vi "q4 character count.vi"() -> ()   [LabVIEW 2025]
panel:
  out "length without spaces":dbl
  out "text":string
  out "length":i32
  in  "Path":path
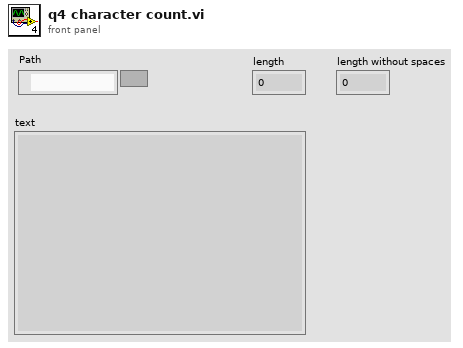
[diagram p1: front panel]
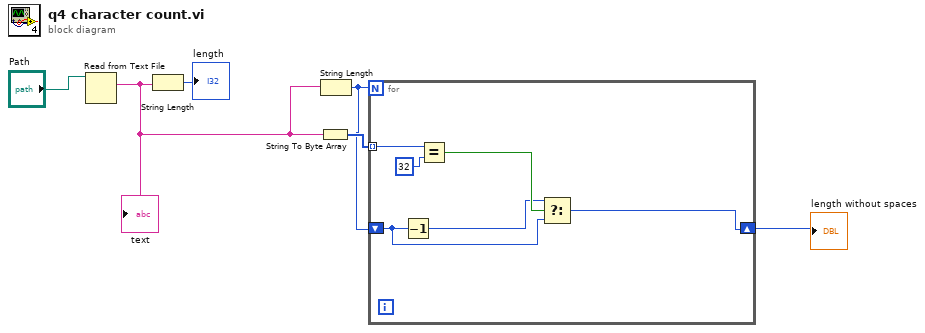
[diagram p0: block diagram]
diagram:
  n1 = Read from Text File(file (use dialog)="Path") -> (text=w2:string)  [unwired: 3 in, 3 out]
  "text" <- w2
  n2 = String Length(string=w2) -> (length=→"length":i32)
  n3 = String To Byte Array(string=w2) -> (unsigned byte array=w4:u8[])
  n4 = String Length(string=w2) -> (length=w1:i32)
  n5 = for {
    N: w1 -> [_]
    tunnel: w4 -> [w12] mode=indexing
    shift-right: [w7] -> w3
    shift-left: w1 -> [w8]
    n6 = Decrement(x=w8) -> (x-1=w9:i32)
    n7 = Equal?(x=w12, y=32) -> (x = y?=w10:bool)
    n8 = Select(t=w9, s=w10, f=w8) -> (s? t:f=w7:i32)
  }
  "length without spaces" <- w3
